vi "Add or Get Property Folder.vi"(6 "Property Folder Name":string, 8 "error in (no error)":errorcluster, 9 "WantsWrite":bool, 10 "WantsRead":bool, 11 "Parent ProjectItem Refnum in":refnum<vi>) -> (0 "error out":errorcluster, 1 "Folder Refnum out":refnum<vi>, 2 "Created?":bool)   [LabVIEW 2021, in "MemberVICreation.lvlib" / "BaseAccessorScripter.lvclass"]
uses:
  <resource>/Framework/Providers/LVClassLibrary/NewAccessors/BaseAccessorScripter/BaseAccessorScripter.lvclass
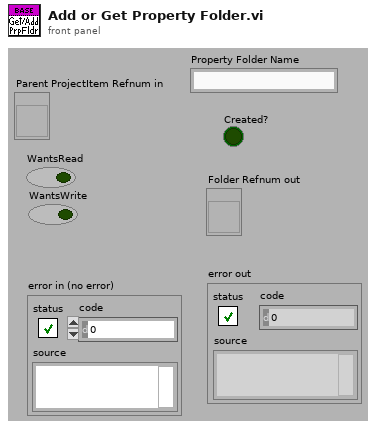
[diagram p1: front panel]
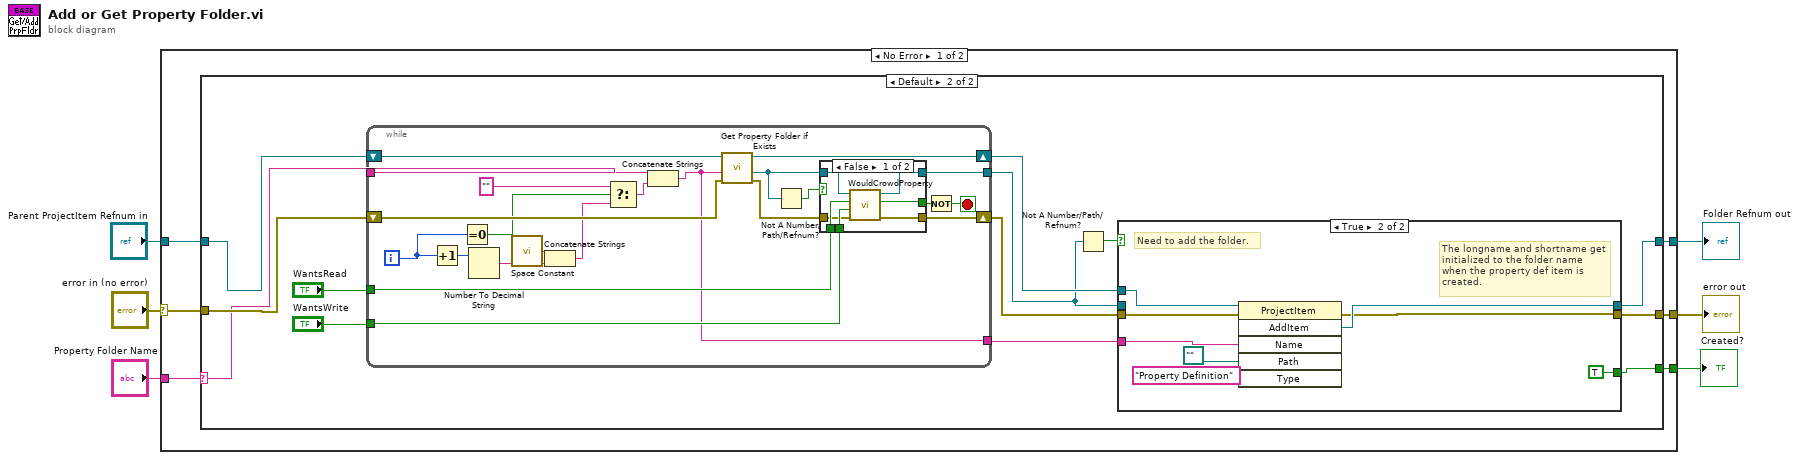
[diagram p0: block diagram]
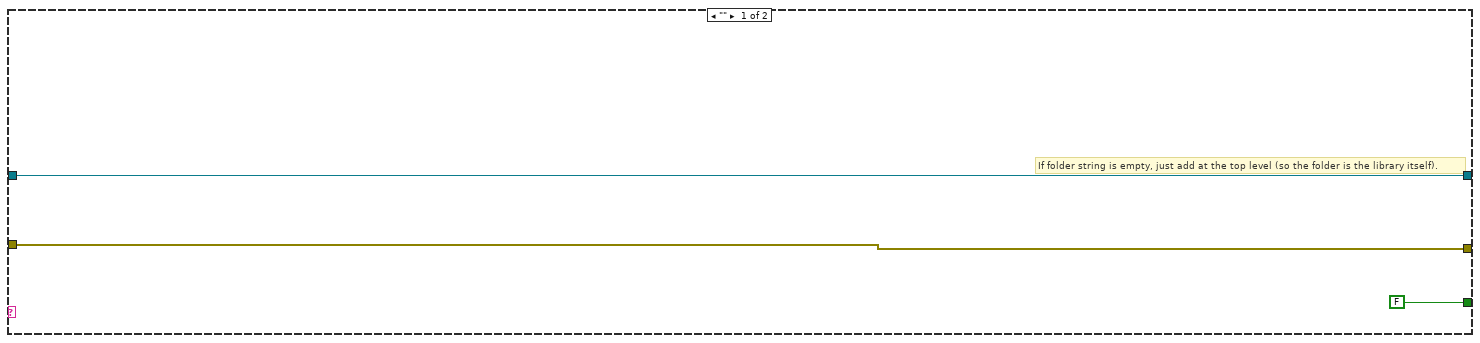
[diagram p2: hidden frame]
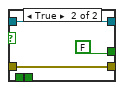
[diagram p3: hidden frame]
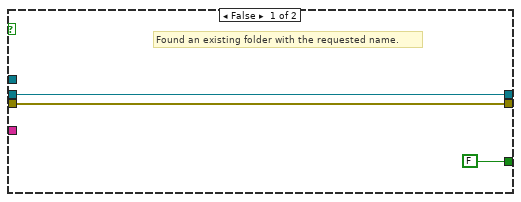
[diagram p4: hidden frame]
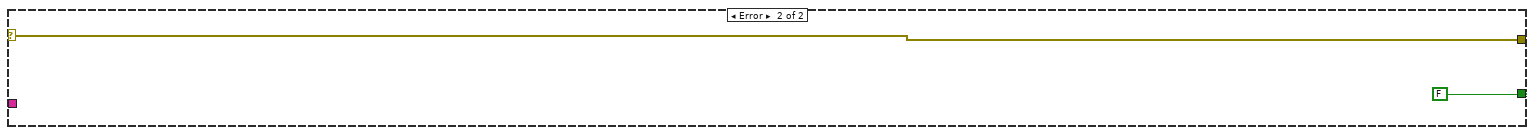
[diagram p5: hidden frame]
diagram:
  n1 = case shown="No Error" "error in (no error)" {
    selector: "error in (no error)" -> [w9 w73]
    tunnel: [w8 w73] -> w5
    tunnel: "Parent ProjectItem Refnum in" -> [w10 _]
    tunnel: "Property Folder Name" -> [w12 _]
    tunnel: [w11 _] -> w2
    tunnel: [w7 FALSE] -> w1
    frame No Error {
      n2 = case shown="Default" w12 {
        selector: w12 -> [_ w21]
        tunnel: [w15 w28] -> w11
        tunnel: w10 -> [w15 w23]
        tunnel: w9 -> [w14 w22]
        tunnel: [w14 w26] -> w8
        tunnel: [FALSE w24] -> w7
        frame "" {
          # "If folder string is empty, just add at the top level (so the folder is the library itself)."
        }
        frame Default {
          n3 = while {
            tunnel: w21 -> [w40]
            tunnel: "WantsWrite" -> [w49]
            tunnel: "WantsRead" -> [w48]
            shift-right: [w45] -> w27
            shift-left: w22 -> [w47]
            shift-right: [w44] -> w25
            shift-left: w23 -> [w50]
            tunnel: [w43] -> w18
            tunnel: [w33] -> w20
            i -> [w38]
            stop <- w42 stop-if-true
            n4 = Increment(x=w38) -> (x+1=w32:i32)
            n5 = Equal To 0?(x=w38) -> (x = 0?=w37:bool)
            n6 = Number To Decimal String(number=w32) -> (decimal integer string=w31:string)  [unwired: 1 in]
            n7 = call <vilib>:"Space Constant.vi"() -> ("String"=w30:string)
            n8 = Concatenate Strings(w30, w31) -> (w29:string)
            n9 = Select(t="" ("Proposed Property Folder Name"), s=w37, f=w29) -> (s? t:f=w36:string)
            n10 = Concatenate Strings(w40, w36) -> (w33:string)
            n11 = call <resource>:"Get Property Folder if Exists.vi"("error in (no error)"=w47, "Property Folder Name"=w33, "Parent ProjectItem Refnum in"=w50) -> ("error out"=w46:errorcluster, "Folder Refnum out"=w34:refnum<vi>, "Parent ProjectItem Refnum out"=w44:refnum<vi>)  [unwired: 6 in]
            n12 = Not A Number/Path/Refnum?(number/path/refnum=w34) -> (NaN/Path/Refnum?=w35:bool)
            n13 = case shown="False" w35 {
              tunnel: w34 -> [w57 w60]
              tunnel: w49 -> [w56 _]
              tunnel: w48 -> [w55 _]
              tunnel: w46 -> [w54 w58]
              tunnel: [w53 w58] -> w45
              tunnel: [w52 w60] -> w43
              tunnel: [w51 FALSE ("Would crowd?")] -> w41
              frame False {
                n14 = call <resource>:"WouldCrowdProperty.vi"("error IO"=w54, "Wants Write"=w56, "WantsRead"=w55, "Proposed Folder Refnum in"=w57) -> ("error out"=w53:errorcluster, "Would crowd?"=w51:bool, "Folder Refnum out"=w52:refnum<vi>)  [unwired: 5 in]
              }
              frame True {
              }
            }
            n15 = Not(x=w41) -> (.not. x?=w42:bool)
          }
          n16 = Not A Number/Path/Refnum?(number/path/refnum=w18) -> (NaN/Path/Refnum?=w19:bool)
          n17 = case shown="True" w19 {
            tunnel: w25 -> [_ w68]
            tunnel: [w62 w65] -> w28
            tunnel: w20 -> [_ w66]
            tunnel: w27 -> [w63 w70]
            tunnel: [w63 w64] -> w26
            tunnel: w18 -> [w62 _]
            tunnel: [FALSE TRUE] -> w24
            frame False {
              # "Found an existing folder with the requested name."
            }
            frame True {
              # "The longname and shortname get initialized to the folder name when the property def item is created."
              # "Need to add the folder."
              n18 = invoke class="ProjectItem" method="AddItem"(reference=w68, error in=w70, "Name"=w66, "Path"=path "", "Type"="Property Definition") -> (error out=w64:errorcluster, "AddItem"=w65:refnum<vi>)  [unwired: 1 in, 4 out]
            }
          }
        }
      }
    }
    frame Error {
    }
  }
  "error out" <- w5
  "Folder Refnum out" <- w2
  "Created?" <- w1
